vi "Init_event.vi"(8 "error in (no error)":errorcluster, 9 "response event":T1, 10 "Name":string, 11 "EventResponder in":refnum<class "EventResponder.lvclass">) -> (0 "error out":errorcluster, 3 "EventResponder out":refnum<class "EventResponder.lvclass">)   [LabVIEW 2013, in "EventResponder.lvclass"]
doc: "Initializes an instance of the EventResponder class"
uses:
  EventResponder.lvclass
  response_event.ctl
  response.ctl
  driver_status.ctl
  EventResponder.lvclass/EventResponder.ctl
  BaseResponder/BaseResponder.lvclass
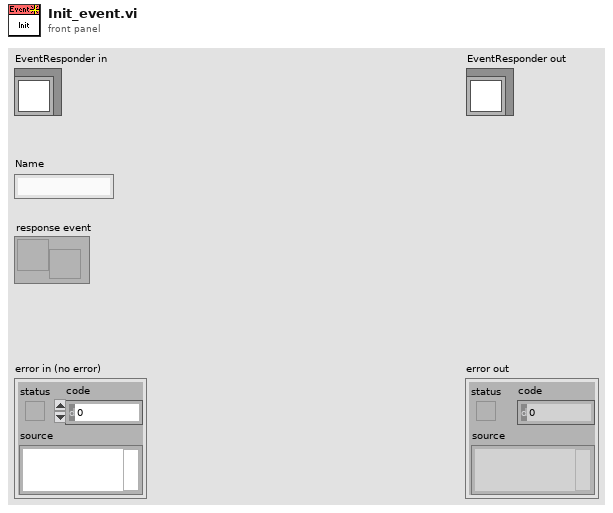
[diagram p1: front panel]
types:
  T1 = typedef "response_event.ctl" = refnum<user-event>
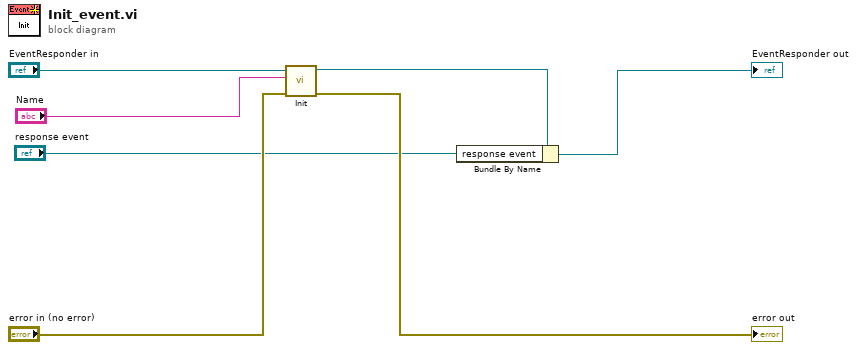
[diagram p0: block diagram]
diagram:
  n1 = call "Init.vi"("error in (no error)"="error in (no error)", "Name"="Name", "BaseResponder in"="EventResponder in") -> ("error out"=→"error out":errorcluster, "BaseResponder out"=w1:refnum<class "EventResponder.lvclass">)  [unwired: 7 in]
  n2 = Bundle By Name(cluster=w1, "response event"="response event") -> (→"EventResponder out":refnum<class "EventResponder.lvclass">)
